vi "main_v20.vi"() -> ()   [LabVIEW 2016]
uses:
  <vilib>/Utility/file.llb/Write Delimited Spreadsheet (DBL).vi
  <vilib>/addons/database/Connection.llb/DB Tools Open Connec (Path).vi
  <vilib>/addons/database/Auxilliary.llb/DB Tools Format Datetime String (Time Stamp).vi
  <vilib>/addons/database/NI_Database_API.lvlib
panel:
  out "error out":errorcluster={"status"=FALSE, "code"=1073676418, "source"="VISA Close in N5700 Close.vi->main_v17.vi"}
  in  "Tab Control":T1(tab)
  out "Status_output_DC 2":bool caption="Ligado"
  out "Status_PS":bool caption="Conexão"
  out "Status_output_DC":bool caption="Ligado"
  out "Status_DC":bool caption="Conexão"
  out "battery_name 3":string="Manual" caption="Bateria Selecionada"
  in  "Historic_page":bool
  in  "graph_page":bool
  in  "Battery_page":bool
  in  "Test_page":bool
  in  "Charge_page":bool
  in  "Exit1":bool
  in  "Cap_nom":dbl caption="Capacidade Nominal (Ah)"
  in  "padrao_cap":dbl caption="Padrão Capacidade (h)"
  in  "Tensao_carga":dbl caption="Tensão Carga (V)"
  in  "corrente_res":dbl caption="Corrente Residual (A)"
  in  "SOC":dbl caption="Estado de Carga (%)"
  in  "corrente_max":dbl caption="Corrente de Carga (A)"
  in  "Tensao_corte":dbl caption="Tensão de Corte (V)"
  in  "ok_refresh_soc":bool
  in  "refresh_soc":bool
  in  "Charge_page2":bool
  in  "Test_page2":bool
  in  "New_battery":bool
  in  "Exit2":bool
  in  "Home1":bool
  out "data bateria":string[][](table)
  in  "Ativar Banco":bool
  in  "Table ID":u16(ring) items=["Bateria Unipower 1", "Bateria Unipower 2", "Bateria Unipower 3", "Bateria Unipower 4", "Bateria Unipower 5", "Bateria Unipower 6", "Bateria Unipower 7", "Bateria Unipower 8", "Bateria Litio 3 em serie"]
  in  "data_soc":cluster{"soc_db":dbl}={"soc_db"=100.0}
  in  "data insert":T2={"Descrição"="Descrição", "cap_db"=0.0, "tensao_nom_db"=0.0, "tensao_carg_db"=0.0, "corr_carg_db 2"=0.0, "tensao_corte_db"=0.0, "corr_res_db"=0.0, "soc_db"=0.0}
  in  "Exit3":bool
  in  "Home3":bool
  in  "Insert_battery":bool
  in  "Table ID 3":u16(ring) items=["Capacidade Nominal (Ah)", "Resistência Interna (ohm)", "Corrente de Curto-Circuito (A)"]
  in  "Table ID 2":u16(ring) items=["Bateria Unipower 1", "Bateria Unipower 2", "Bateria Unipower 3", "Bateria Unipower 4", "Bateria Unipower 5", "Bateria Unipower 6", "Bateria Unipower 7", "Bateria Unipower 8", "Bateria Litio 3 em serie"]
  out "data ensaio":string[][](table)
  in  "Exit4":bool
  in  "Home2":bool
  out "data bateria 2":string[][](table)
  in  "battery_select":bool
  in  "graph_select":bool
  in  "Exit5":bool
  in  "Home4":bool
  out "SoC_charge":dbl caption="Estado de Carga"
  out "Timer_charge":dbl caption="Tempo"
  out "Output_Current":dbl caption="Corrente"
  out "Output_Voltage":dbl caption="Tensão"
  out "Charge Active":bool
  in  "Radio Buttons":enum32{"Carga TC", "Carga CC"}(radio) caption="Modo de Carga"
  out "Current_Limit":dbl caption="Corrente"
  out "Voltage_Limit":dbl caption="Tensão"
  in  "Output On (T)":bool
  in  "auxiliar 2":bool
  out "battery_name 2":string="Manual" caption="Bateria Selecionada"
  out "soc_ensaio":dbl caption="Estado de Carga"
  out "Timer_ensaio":dbl caption="Tempo"
  out "DC_Current":dbl caption="Corrente"
  out "DC_Voltage":dbl caption="Tensão"
  in  "Start":bool
  out "CC Active":bool
  in  "battery_select2":bool
  in  "graph_select2":bool
  out "battery_name":string="Manual" caption="Bateria Selecionada"
  in  "Ensaios":u16(ring) items=["Capacidade Regime Nominal", "Capacidade Diferente de Regime Nominal", "Resistência Interna", "Ciclos de carga e descarga", "Caracterização"]
  in  "Exit6":bool
  in  "cap_soc":dbl caption="Capacidade"
  in  "info_ensaio":enum32{"1", "2", "3", "4", "5"}(tab)
  out "padrao_cap2":dbl caption="Padrão Capacidade (h)"
  out "cap_bat":dbl caption="Capacidade (Ah)"
  out "cap_nom_ensaio":dbl caption="Capacidade Real (Ah)"
  in  "aux_cap_ensaio":bool
  in  "aux_soc_ensaio1":bool
  out "cap_fn_calc":dbl caption="Capacidade Real (Ah)"
  in  "cap_fn":dbl caption="Capacidade (Ah)"
  in  "corr_fn":dbl caption="Corrente (A)"
  out "res_cap":dbl caption="Capacidade (Ah)"
  out "res_ensaio":dbl caption="Resistência (ohm)"
  out "curto_ensaio":dbl caption="Corrente Curto-Circuito (A)"
  out "res_volt_1":dbl caption="Volt_res_1"
  out "res_curr_1":dbl caption="Corr_res_1"
  out "res_curr_2":dbl caption="Corr_res_2"
  out "res_volt_2":dbl caption="Volt_res_2"
  in  "aux_res_ensaio":bool
  in  "aux_soc_ensaio2":bool
  in  "curr_carac":dbl caption="Corrente"
  in  "twait":dbl caption="Tempo Relax"
  in  "cap_caract":dbl caption="Capacidade"
  in  "pulso_soc":dbl caption="Pulso SoC"
  out "cont_pulso":dbl caption="Contador Pulso"
  out "est_time":dbl caption="Tempo Estimado"
  out "COP":bool
  in  "tinicio":dbl caption="T inicio"
  out "tpulso":dbl caption="Tempo Descarga"
  in  "Home5":bool
  out "cap_ensaio":dbl caption="Capacidade"
  in  "aux_soc":bool
  out "WFC Current Load":dbl(graph)=0.007083870470523834
  out "WFC Voltage Load":dbl(graph)=12.54011344909668
  out "Waveform Chart Voltage":dbl(graph)=12.56
  out "Waveform Chart Current":dbl(graph)
  in  "back_charge":bool
  in  "back_ens":bool
  in  "Home6":bool
  in  "Exit7":bool
  # "MENU"
  # "Desenvolvido por William Rocha"
  # "Deseja ativar o banco de dados?"
  # "BATERIAS"
  # "Desenvolvido por William Rocha"
  # "REGISTRAR BATERIA"
  # "Desenvolvido por William Rocha"
  # "Desenvolvido por William Rocha"
  # "MOSTRAR BATERIAS"
  # "Instruções"
  # "Para iniciar o ensaio de capacidade siga o procedimento de abaixo:\n  1 - Verifique se a bateria está conectada aos equipamentos  \n  2 - Verifique a bateria selecionada no banco de dados ou insira os dados manualmente  \n  3 - Selecione o modo de carga\n  4 - Pressione o botão iniciar carga\n\n  A carga é finalizada ao atingir 100 % do estado de carga. A carga pode ser encerrada em qualquer momento pelo usuário da carga."
  # "Desenvolvido por William Rocha"
  # "RECARGA"
  # "V"
  # "A"
  # "%"
  # "s"
  # "Iniciar Carga"
  # "Configuração"
  # "V"
  # "A"
  # "Modo de  Carga"
  # "Medições"
  # "Iniciar Ensaio"
  # "Medições"
  # "V"
  # "A"
  # "Ensaio Ativo"
  # "%"
  # "s"
  # "Instruções"
  # "Para iniciar o ensaio siga o procedimento de abaixo:\n  1 - Verifique se a bateria está conectada aos equipamentos\n  2 - Verifique a bateria selecionada no banco de dados ou insira os dados manualmente \n  3 - Pressione o botão iniciar carga\n  4 - Espere até o fim do ensaio para obter o resultado\n\n  O ensaio é finalizado automaticamente e o resultado será inserido no banco de dados, caso o mesmo esteja ativado. Porém, o ensaio pode ser encerrado em qualquer momento pelo usuário e o resultado não será contabalizado."
  # "ENSAIOS"
  # "Desenvolvido por William Rocha"
  # "Fonte CC"
  # "Carga Eletrônica"
  # "Desenvolvido por William Rocha"
  # "Gráficos"
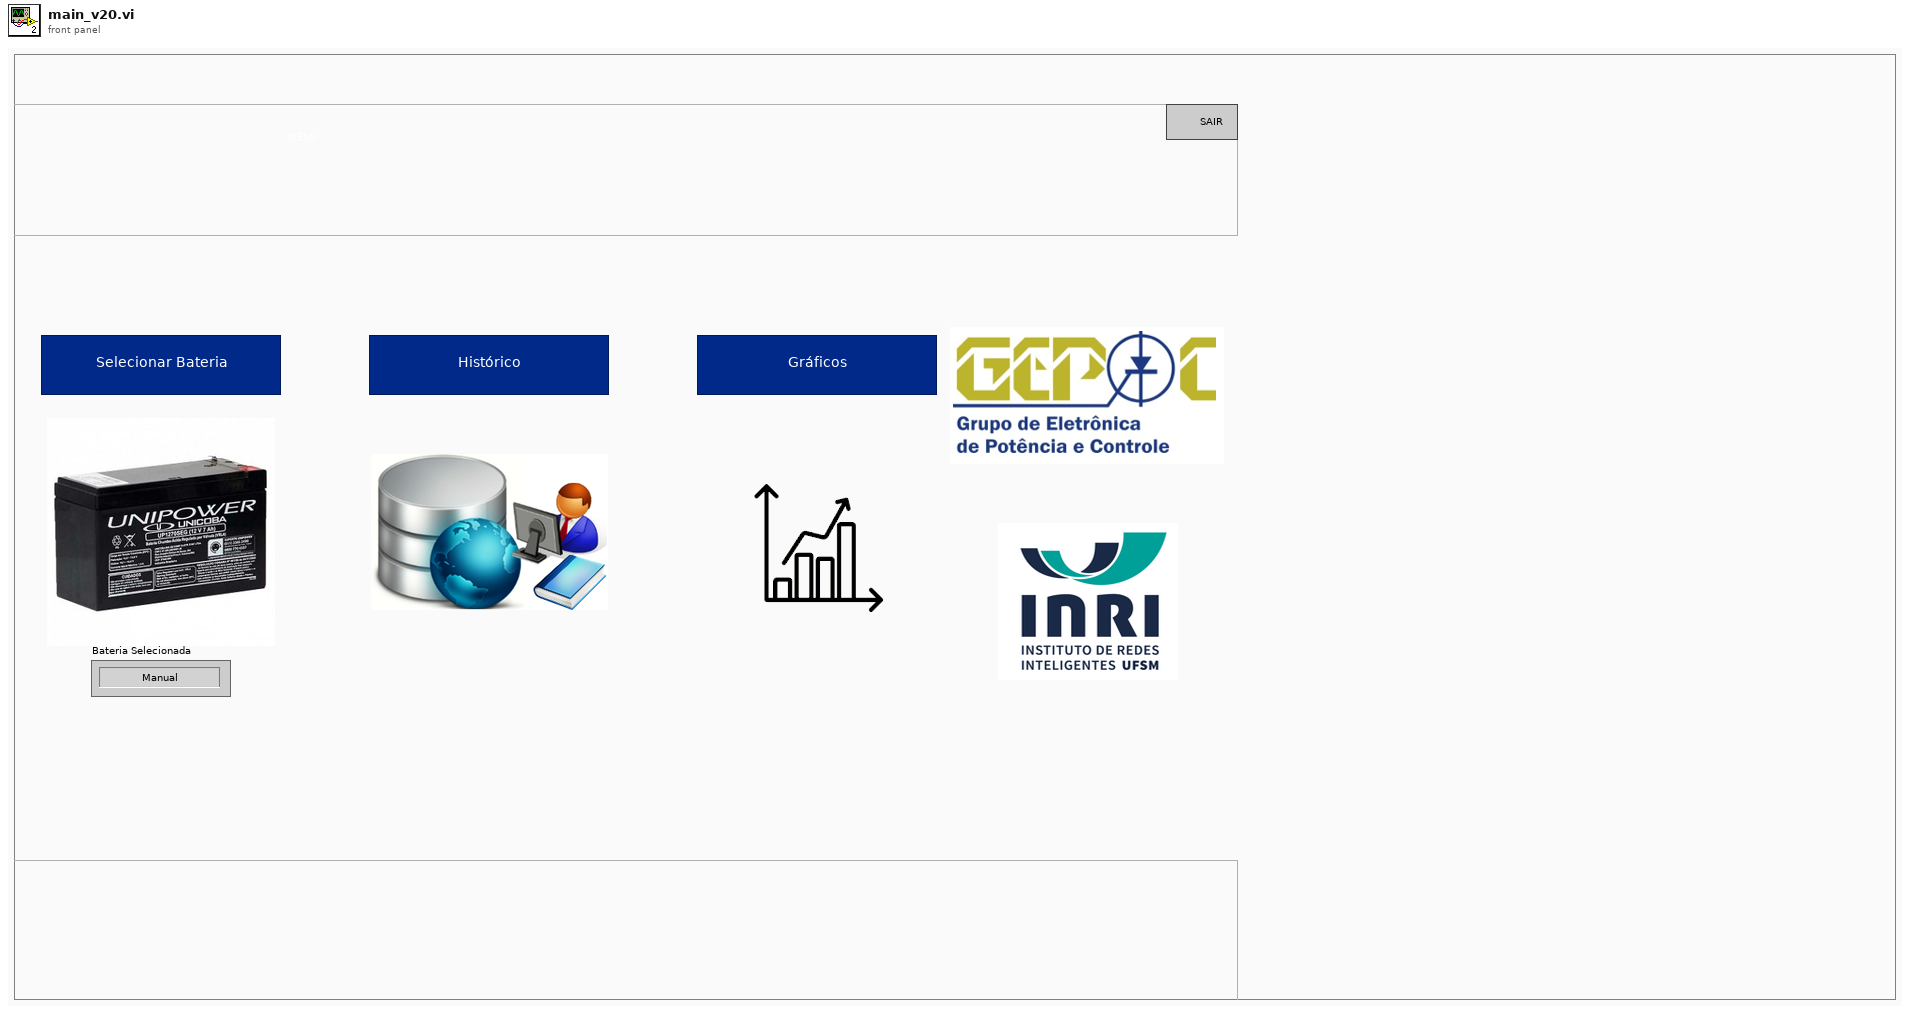
[diagram p1: front panel]
types:
  T1 = enum32{"Home", "Battery Page", "Register Battery Page", "Show battery page", "Charge Page", "Test Page", "Graphs"}
  T2 = cluster{"Descrição":string, "cap_db":dbl, "tensao_nom_db":dbl, "tensao_carg_db":dbl, "corr_carg_db 2":dbl, "tensao_corte_db":dbl, "corr_res_db":dbl, "soc_db":dbl}
  T3 = enum32{"Home", "Battery Page", "Register Battery Page", "Show battery page", "Charge Page", "Test Page"}
  T4 = typedef "NI_Database_API.lvlib/Conn ObjectReference.ctl" = refnum<k1>
  T5 = cluster{"Table ID":u16, "date/time string":string, i32, "cap_nom_ensaio":dbl}
  T6 = cluster{"Table ID":u16, "date/time string":string, i32, "res_ensaio":dbl}
  T7 = cluster{"Table ID":u16, "date/time string":string, i32, "curto_ensaio":dbl}
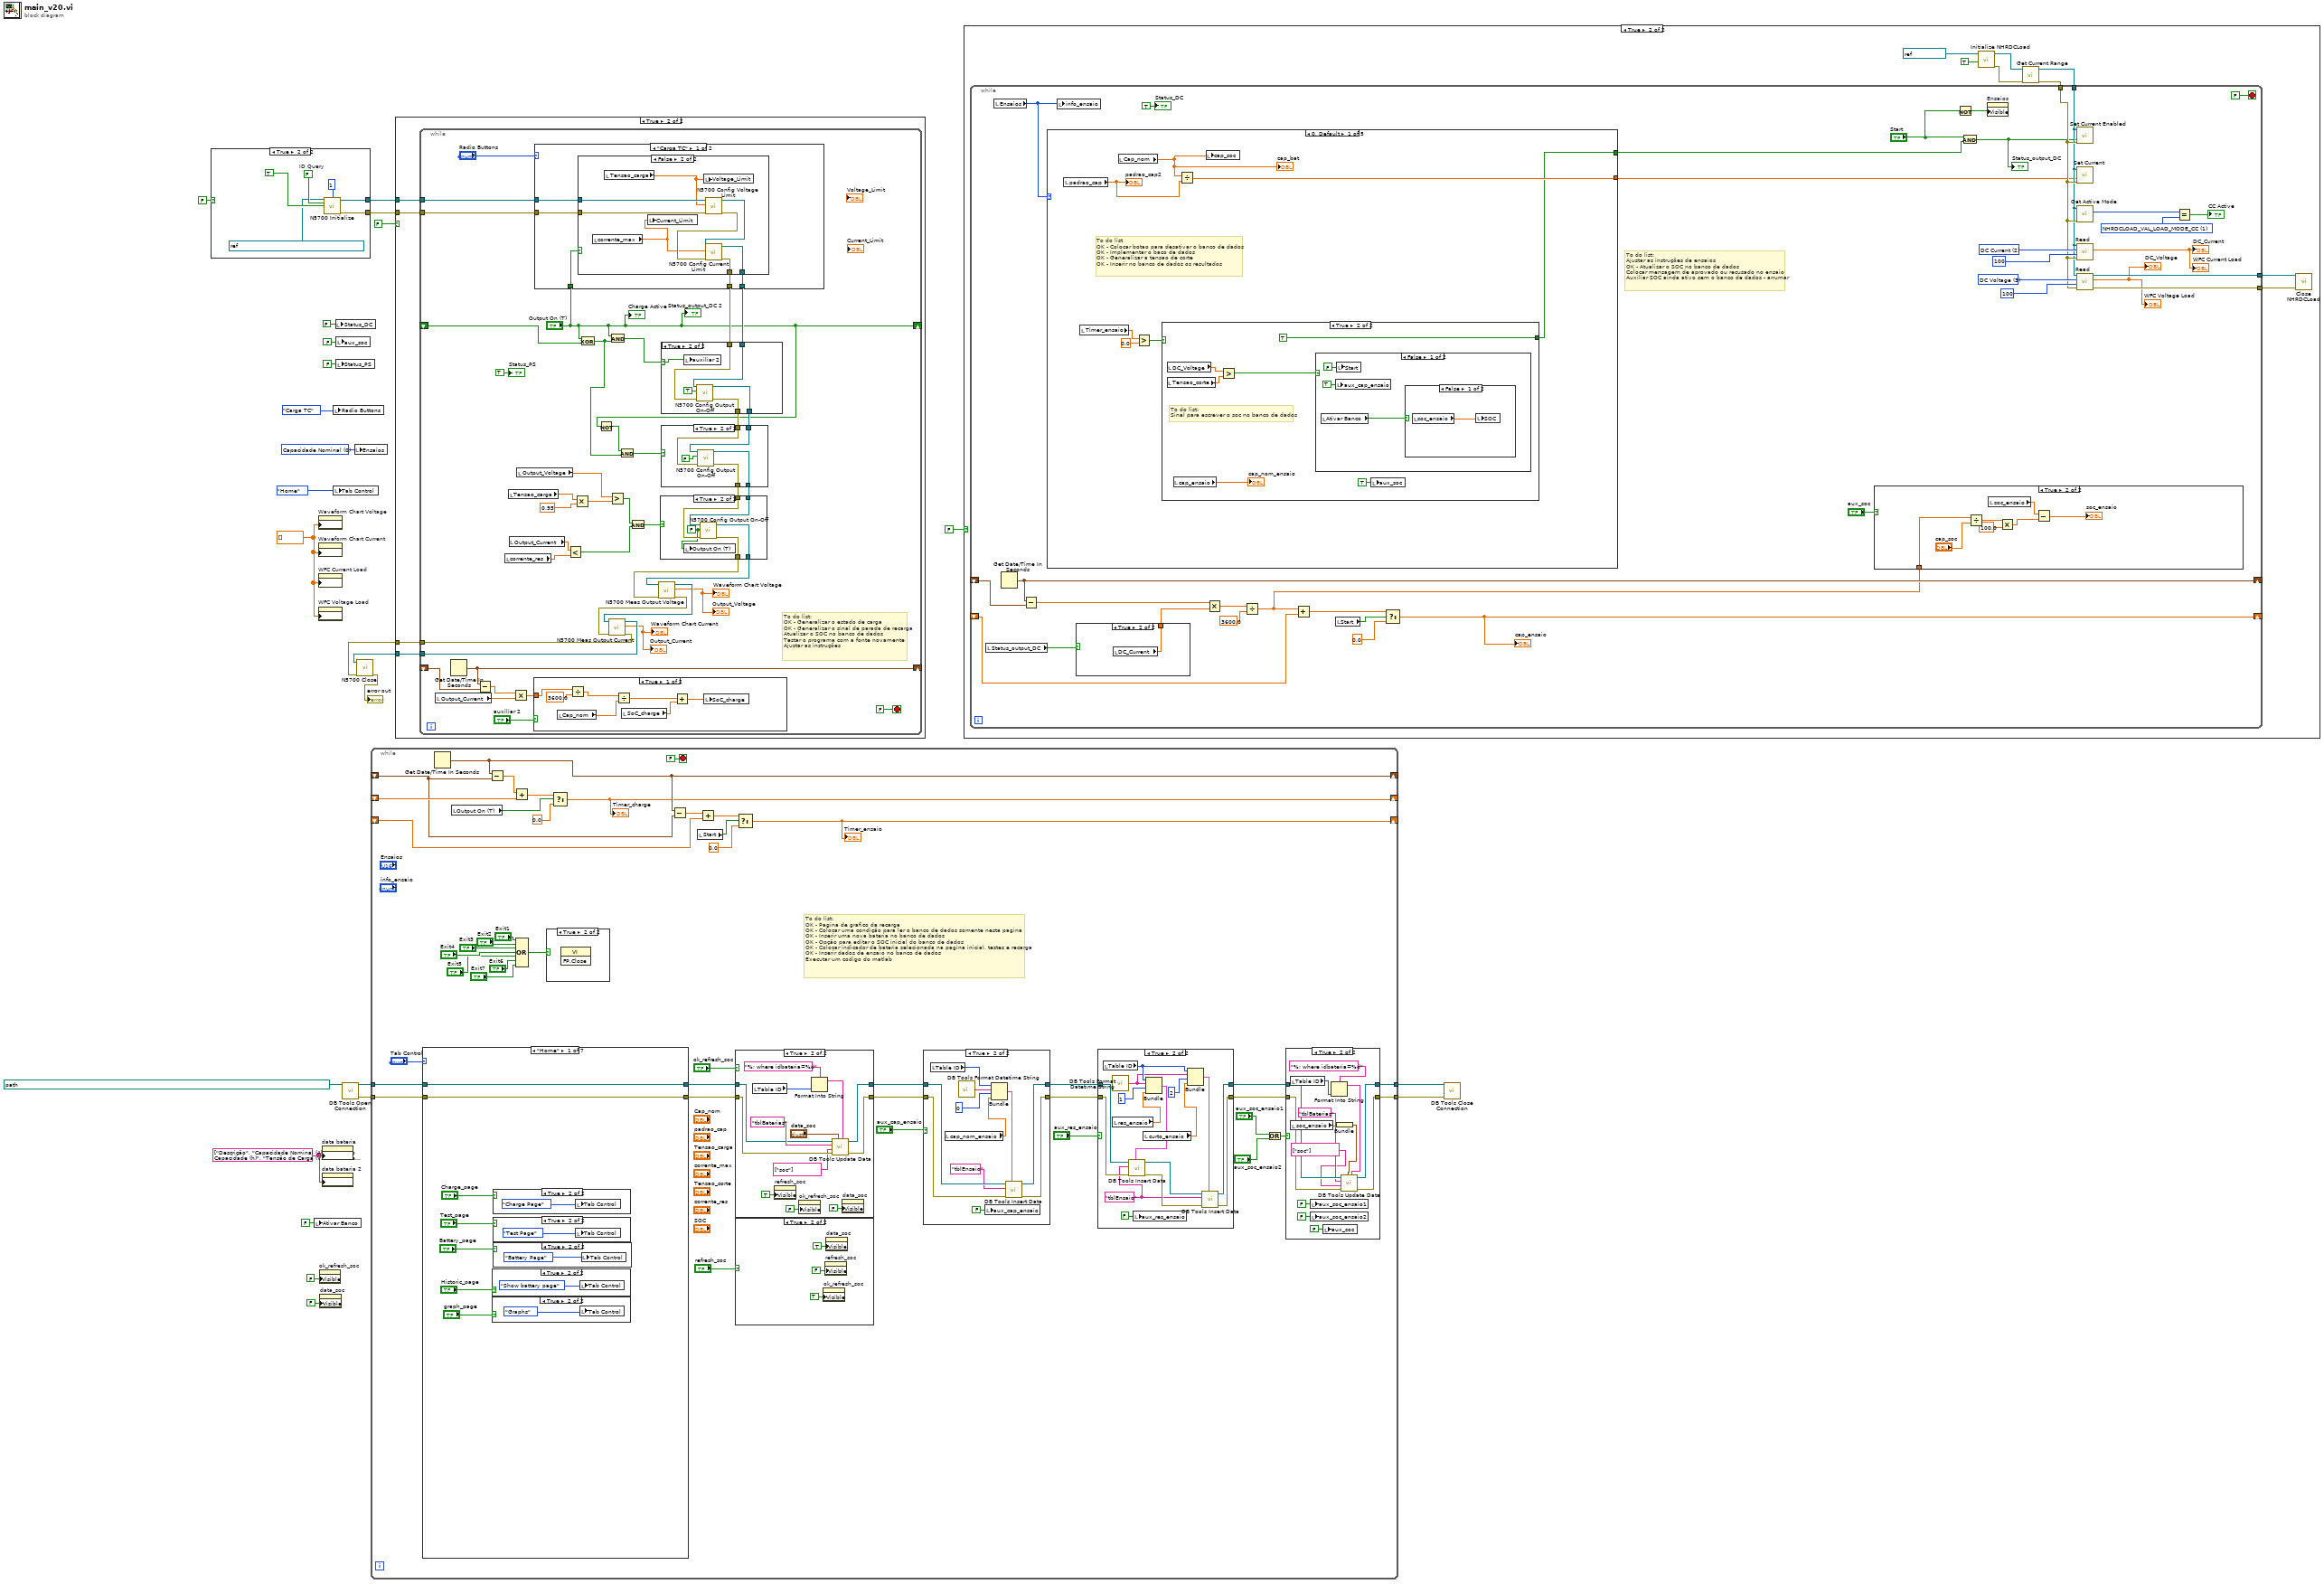
[diagram p0: block diagram]
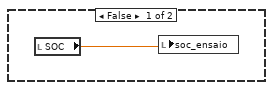
[diagram p4: hidden frame]
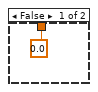
[diagram p5: hidden frame]
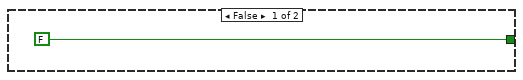
[diagram p6: hidden frame]
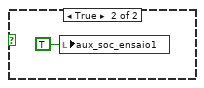
[diagram p7: hidden frame]
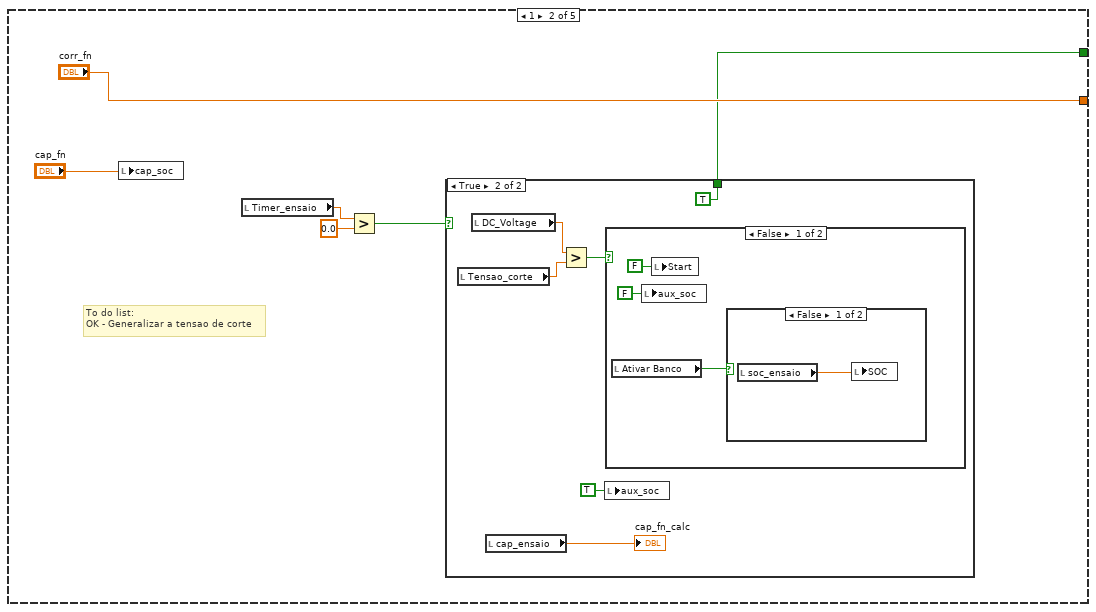
[diagram p9: hidden frame]
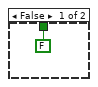
[diagram p10: hidden frame]
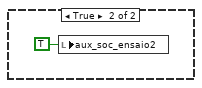
[diagram p11: hidden frame]
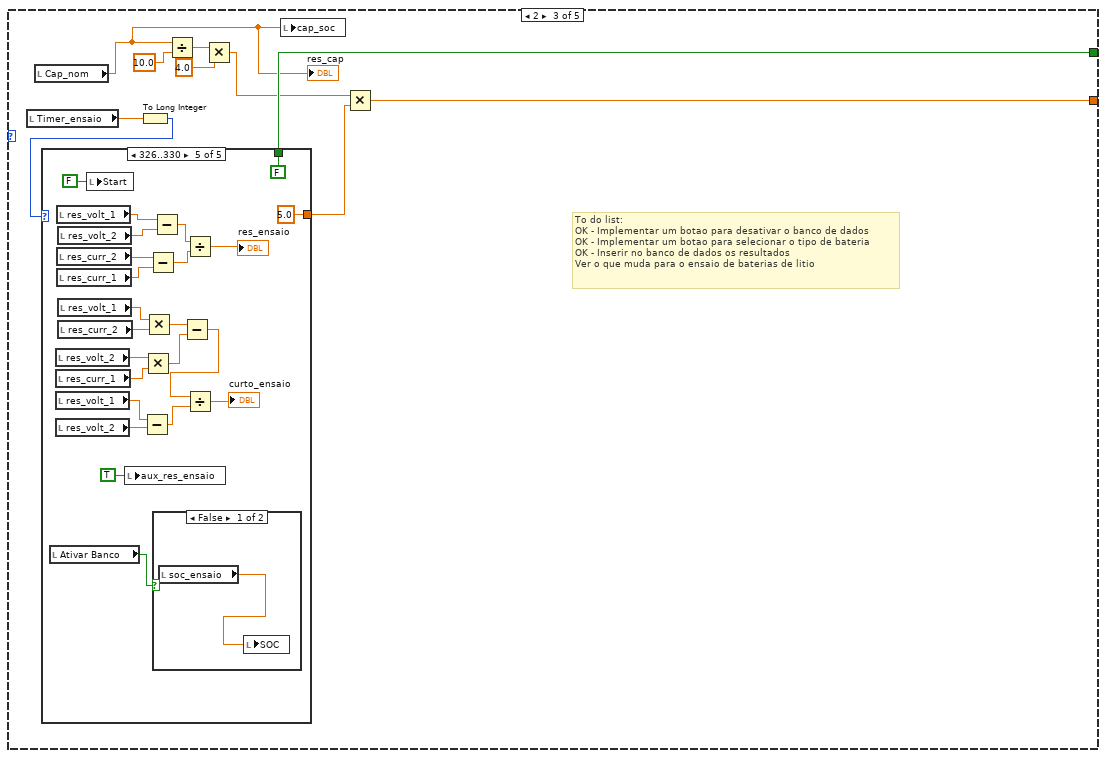
[diagram p13: hidden frame]
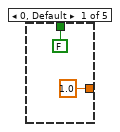
[diagram p14: hidden frame]
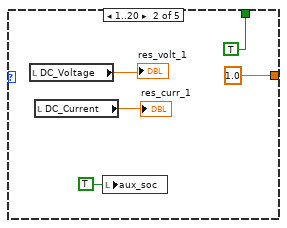
[diagram p15: hidden frame]
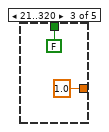
[diagram p16: hidden frame]
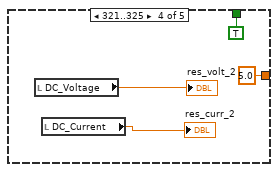
[diagram p17: hidden frame]
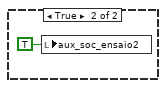
[diagram p18: hidden frame]
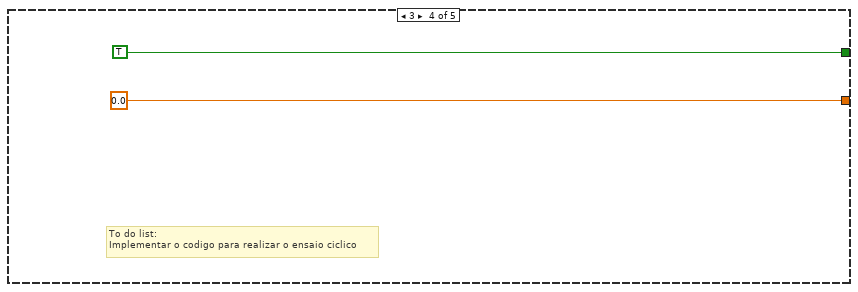
[diagram p19: hidden frame]
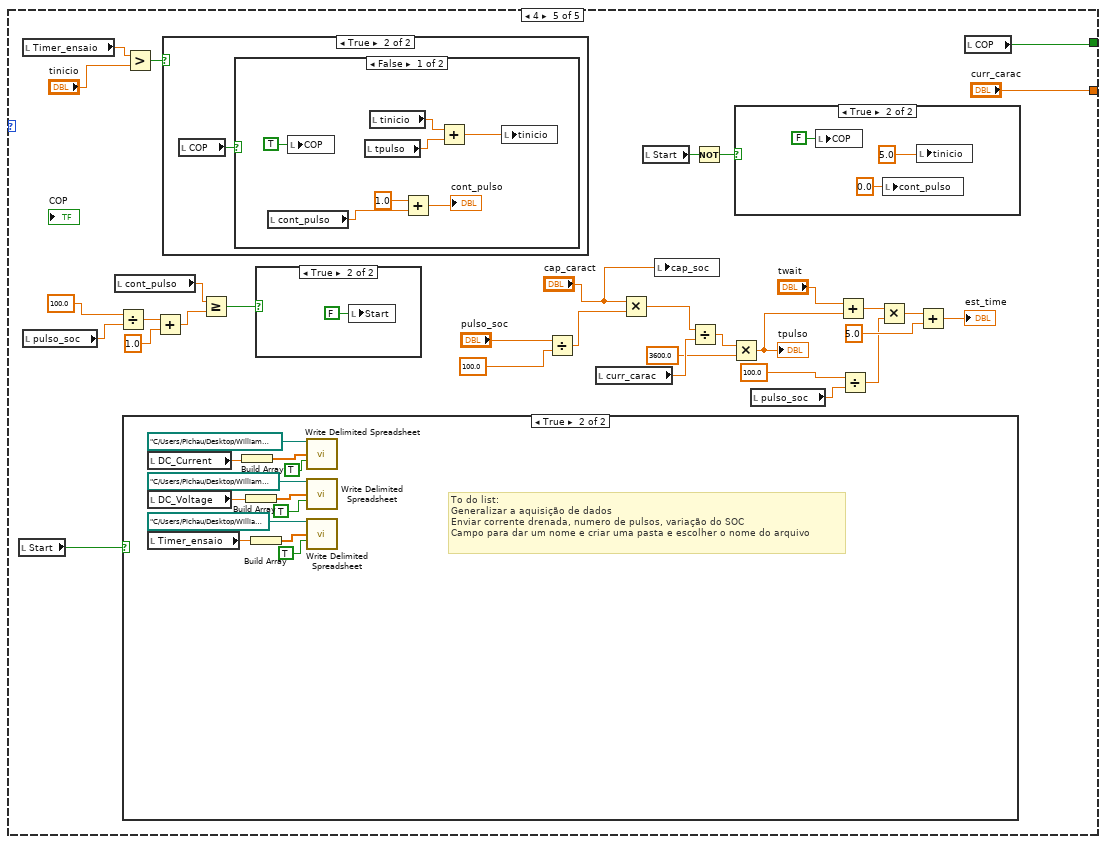
[diagram p20: hidden frame]
diagram:
  w6 = string[] ["Descrição", "Capacidade Nominal (Ah)", "Padrão Capacidade (h)", "Tensão de Carga (V)", "Corrente Máxima (A)", "Tensão de Corte (V)", "Corrente Residual (A)", "SOC (%)"] ("columns")
  w14 = u16 0 items=["Capacidade Nominal"] ("Table ID")
  w10 = dbl[] [] ("History Data")
  n1 = case shown="True" FALSE {
    tunnel: [_ w25] -> w23
    tunnel: [_ w27] -> w20
    frame False {
    }
    frame True {
      w29 = FALSE  # ID Query
      n2 = call <instrlib>:"N5700 Initialize.vi"("VISA name"=refnum<visa-resource-name> "TCPIP0::A-N8762A-1651P.local::inst0::INSTR", "Timeout (3 sec)"=u32 1, "ID Query (T)"=w29, "Reset (T)"=TRUE ("Reset (F)")) -> ("VISA out"=w25:refnum<visa-resource-name>, "error out"=w27:errorcluster)  [unwired: 10 in]
    }
  }
  n3 = local write "Ativar Banco"(FALSE ("Ativar Banco")) -> ()
  n4 = property on="Waveform Chart Voltage" class="WFChart (strict)"("History Data"=w10) -> ()  [unwired: 2 in, 2 out]
  n5 = property on="Waveform Chart Current" class="WFChart (strict)"("History Data"=w10) -> ()  [unwired: 2 in, 2 out]
  n6 = property on="WFC Current Load" class="WFChart (strict)"("History Data"=w10) -> ()  [unwired: 2 in, 2 out]
  n7 = property on="WFC Voltage Load" class="WFChart (strict)"("History Data"=w10) -> ()  [unwired: 2 in, 2 out]
  n8 = property on="ok_refresh_soc" class="Bool"("Visible"=FALSE) -> ()  [unwired: 2 in, 2 out]
  n9 = property on="data_soc" class="Clust (strict)"("Visible"=FALSE) -> ()  [unwired: 2 in, 2 out]
  n10 = property on="data bateria" class="Tbl (strict)"("Column Headers[]"=w6) -> ()  [unwired: 2 in, 2 out]
  n11 = property on="data bateria 2" class="Tbl (strict)"("Column Headers[]"=w6) -> ()  [unwired: 2 in, 2 out]
  n12 = local write "Radio Buttons"(enum32{"Carga TC", "Carga CC"}."Carga TC" ("Radio Buttons")) -> ()
  n13 = local write "Tab Control"(T3."Home" ("Tab Control")) -> ()
  n14 = local write "Status_DC"(FALSE ("Status_DC")) -> ()
  n15 = local write "aux_soc"(FALSE ("aux_soc")) -> ()
  n16 = local write "Status_PS"(FALSE ("Status_PS")) -> ()
  n17 = call-poly <vilib>:"DB Tools Open Connection.vi"("connection information"=path "D:/UFSM/Engenharia de Controle e Automação/9 Semestre/Trabalho de Conclusão de Curso “A” – DPEE 1046/TCC/TCC - William Rochav5/database/database2_2.udl") -> ("error out"=w7:errorcluster, "connection reference"=w8:T4)  [unwired: 7 in]
  n18 = local write "Ensaios"(w14) -> ()
  n19 = while {
    shift-right: [w66] -> _
    shift-left: _ -> [w65]
    shift-right: [w59] -> _
    shift-left: _ -> [w72]
    shift-right: [w58] -> _
    shift-left: _ -> [w61]
    tunnel: w8 -> [w49]
    tunnel: w7 -> [w48]
    tunnel: [w37] -> w5
    tunnel: [w35] -> w4
    stop <- FALSE stop-if-true
    # "To do list:\nOK - Pagina de grafico da recarga\nOK - Colocar uma condição para ler o banco de dados somente nesta pagina\nOK - Inserir uma nova bateria no banco de dados\nOK - Opção para editar o SOC inicial do banco de dados\nOK - Colocar indicador de bateria selecionada na pagina inicial, testes e recarga\nOK - Inserir dados de ensaio no banco de dados\nExecutar um codigo do matlab"
    n20 = case shown="\"Home\"" "Tab Control" {
      tunnel: [w140 w157 w216 w236 w254 w262 w270] -> w47
      tunnel: w49 -> [w140 w160 w217 w239 w254 w262 w270]
      tunnel: [w139 w158 w215 w237 w253 w261 w269] -> w46
      tunnel: w48 -> [w139 w159 w218 w238 w253 w261 w269]
      frame "Home" {
        n21 = case shown="True" "Historic_page" {
          frame False {
          }
          frame True {
            n22 = local write "Tab Control"(T3."Show battery page" ("Tab Control")) -> ()
          }
        }
        n23 = case shown="True" "graph_page" {
          frame False {
          }
          frame True {
            n24 = local write "Tab Control"(T1."Graphs" ("Tab Control")) -> ()
          }
        }
        n25 = case shown="True" "Charge_page" {
          frame False {
          }
          frame True {
            n26 = local write "Tab Control"(T3."Charge Page" ("Tab Control")) -> ()
          }
        }
        n27 = case shown="True" "Test_page" {
          frame False {
          }
          frame True {
            n28 = local write "Tab Control"(T3."Test Page" ("Tab Control")) -> ()
          }
        }
        n29 = case shown="True" "Battery_page" {
          frame False {
          }
          frame True {
            n30 = local write "Tab Control"(T3."Battery Page" ("Tab Control")) -> ()
          }
        }
      }
      frame "Battery Page" {
        n31 = Not(x="Ativar Banco") -> (.not. x?=w151:bool)
        n32 = case shown="True" "Ativar Banco" {
          tunnel: w160 -> [w171 w207]
          tunnel: w159 -> [w170 w206]
          tunnel: [w171 w203] -> w157
          tunnel: [w170 w202] -> w158
          frame False {
            w166 = FALSE ("Visible")
            w169 = "Manual" ("battery_name")
            n33 = property on="New_battery" class="Bool"("Visible"=FALSE) -> ()  [unwired: 2 in, 2 out]
            n34 = property on="data_soc" class="Clust (strict)"("Visible"=w166) -> ()  [unwired: 2 in, 2 out]
            n35 = property on="refresh_soc" class="Bool"("Visible"=FALSE) -> ()  [unwired: 2 in, 2 out]
            n36 = property on="ok_refresh_soc" class="Bool"("Visible"=FALSE) -> ()  [unwired: 2 in, 2 out]
            n37 = property on="Table ID" class="Ring (strict)"("Visible"=w166) -> ()  [unwired: 2 in, 2 out]
            "battery_name" <- w169
            "battery_name 2" <- w169
            "battery_name 3" <- w169
          }
          frame True {
            w173 = TRUE ("Visible")
            n38 = call <vilib>:"DB Tools Select All Data.vi"("error in (no error)"=w206, "columns"=string[] ["Descricao", "capacidade", "padrao_cap", "tensao_carga", "corrente", "tensao_corte", "corrente_res", "soc"], "table"="tblBaterias", "connection reference"=w207) -> ("error out"=w202:errorcluster, "data"=w177:string[][], "connection reference out"=w203:T4)  [unwired: 2 in]
            "data bateria" <- w177
            n39 = Index Array(array=w177, index (row)="Table ID", index (col)=1 ("disabled index (col)")) -> (element=w199:string)
            n40 = Index Array(array=w177, index (row)="Table ID", index (col)=2) -> (element=w194:string)
            n41 = Index Array(array=w177, index (row)="Table ID", index (col)=3) -> (element=w193:string)
            n42 = Index Array(array=w177, index (row)="Table ID", index (col)=4 ("disabled index (col)")) -> (element=w183:string)
            n43 = Index Array(array=w177, index (row)="Table ID", index (col)=5 ("disabled index (col)")) -> (element=w184:string)
            n44 = Index Array(array=w177, index (row)="Table ID", index (col)=6 ("disabled index (col)")) -> (element=w185:string)
            n45 = Index Array(array=w177, index (row)="Table ID", index (col)=7 ("disabled index (col)")) -> (element=w186:string)
            n46 = Index Array(array=w177, index (row)="Table ID", index (col)=0 ("disabled index (col)")) -> (element=w174:string)
            n47 = Fract/Exp String To Number(use system decimal point (T)=TRUE, string=w199) -> (number=w197:dbl)  [unwired: 2 in, 1 out]
            n48 = Fract/Exp String To Number(string=w194) -> (number=w192:dbl)  [unwired: 3 in, 1 out]
            n49 = Fract/Exp String To Number(string=w193) -> (number=w191:dbl)  [unwired: 3 in, 1 out]
            n50 = Fract/Exp String To Number(string=w183) -> (number=w182:dbl)  [unwired: 3 in, 1 out]
            n51 = Fract/Exp String To Number(string=w184) -> (number=w181:dbl)  [unwired: 3 in, 1 out]
            n52 = Fract/Exp String To Number(string=w185) -> (number=w179:dbl)  [unwired: 3 in, 1 out]
            n53 = Fract/Exp String To Number(string=w186) -> (number=w180:dbl)  [unwired: 3 in, 1 out]
            n54 = local write "battery_name"(w174) -> ()
            n55 = local write "battery_name 2"(w174) -> ()
            n56 = local write "battery_name 3"(w174) -> ()
            n57 = local write "Tensao_carga"(w191) -> ()
            n58 = local write "corrente_max"(w182) -> ()
            n59 = local write "Tensao_corte"(w181) -> ()
            n60 = local write "Cap_nom"(w197) -> ()
            n61 = local write "padrao_cap"(w192) -> ()
            n62 = local write "corrente_res"(w179) -> ()
            n63 = local write "SOC"(w180) -> ()
            n64 = Index Array(array=w177, index (col)=0) -> (element=w201:string[])  [unwired: 1 in]
            n65 = property on="refresh_soc" class="Bool"("Visible"=w173) -> ()  [unwired: 2 in, 2 out]
            n66 = property on="New_battery" class="Bool"("Visible"=TRUE) -> ()  [unwired: 2 in, 2 out]
            n67 = property on="Table ID" class="Ring (strict)"("Visible"=w173) -> ()  [unwired: 2 in, 2 out]
            n68 = property on="Table ID" class="Ring (strict)"("Strings []"=w201) -> ()  [unwired: 2 in, 2 out]
            n69 = property on="Table ID 2" class="Ring (strict)"("Strings []"=w201) -> ()  [unwired: 2 in, 2 out]
          }
        }
        n70 = property on="data bateria" class="Tbl (strict)"("Visible"="Ativar Banco") -> ()  [unwired: 2 in, 2 out]
        n71 = property on="Cap_nom" class="DigNum (strict)"("Visible"=w151) -> ()  [unwired: 2 in, 2 out]
        n72 = property on="padrao_cap" class="DigNum (strict)"("Visible"=w151) -> ()  [unwired: 2 in, 2 out]
        n73 = property on="Tensao_carga" class="DigNum (strict)"("Visible"=w151) -> ()  [unwired: 2 in, 2 out]
        n74 = property on="corrente_max" class="DigNum (strict)"("Visible"=w151) -> ()  [unwired: 2 in, 2 out]
        n75 = property on="Tensao_corte" class="DigNum (strict)"("Visible"=w151) -> ()  [unwired: 2 in, 2 out]
        n76 = property on="corrente_res" class="DigNum (strict)"("Visible"=w151) -> ()  [unwired: 2 in, 2 out]
        n77 = property on="SOC" class="DigNum (strict)"("Visible"=w151) -> ()  [unwired: 2 in, 2 out]
        n78 = case shown="True" "New_battery" {
          frame False {
          }
          frame True {
            n79 = local write "Tab Control"(T3."Register Battery Page" ("Tab Control")) -> ()
          }
        }
        n80 = case shown="True" "Charge_page2" {
          frame False {
          }
          frame True {
            n81 = local write "Tab Control"(T3."Charge Page" ("Tab Control")) -> ()
          }
        }
        n82 = case shown="True" "Test_page2" {
          frame False {
          }
          frame True {
            n83 = local write "Tab Control"(T3."Test Page" ("Tab Control")) -> ()
          }
        }
        n84 = case shown="True" "Home1" {
          frame False {
          }
          frame True {
            n85 = local write "Tab Control"(T3."Home" ("Tab Control")) -> ()
          }
        }
      }
      frame "Show battery page" {
        n86 = local read "Table ID 3"() -> (w210:u16)
        n87 = property on="Table ID 3" class="Ring (strict)"() -> ("Strings []"=w209:string[])  [unwired: 2 in, 2 out]
        n88 = Index Array(array=w209, index=w210) -> (element=w211:string)
        n89 = case shown="True" "Home2" {
          frame False {
          }
          frame True {
            n90 = local write "Tab Control"(T3."Home" ("Tab Control")) -> ()
          }
        }
        n91 = call <vilib>:"DB Tools Select All Data.vi"("error in (no error)"=w218, "columns"=string[] ["Descricao", "capacidade", "padrao_cap", "tensao_carga", "corrente", "tensao_corte", "corrente_res", "soc"], "table"="tblBaterias", "connection reference"=w217) -> ("error out"=w222:errorcluster, "data"=→"data bateria 2":string[][], "connection reference out"=w221:T4)  [unwired: 2 in]
        n92 = Format Into String(format string="%; where idbateria=%d" ("condition"), "Table ID 2") -> (resulting string=w230:string)  [unwired: 2 in, 1 out]
        n93 = Format Into String(format string="%; and tipo=%d" ("condition"), "Table ID 3") -> (resulting string=w229:string)  [unwired: 2 in, 1 out]
        n94 = Insert Into Array(array=string[] ["Data"], index=1, new element=w211) -> (w214:string[])
        n95 = Concatenate Strings(w230, w229) -> (w231:string)
        n96 = call <vilib>:"DB Tools Select All Data.vi"("optional clause"=w231, "error in (no error)"=w222, "columns"=string[] ["data_ensaio", "valor"], "table"="tblEnsaio", "connection reference"=w221) -> ("error out"=w215:errorcluster, "data"=→"data ensaio":string[][], "connection reference out"=w216:T4)  [unwired: 1 in]
        n97 = property on="data ensaio" class="Tbl (strict)"("Column Headers[]"=w214) -> ()  [unwired: 2 in, 2 out]
      }
      frame "Register Battery Page" {
        n98 = case shown="True" "Home3" {
          frame False {
          }
          frame True {
            n99 = local write "Tab Control"(T3."Home" ("Tab Control")) -> ()
          }
        }
        n100 = case shown="True" "Insert_battery" {
          tunnel: w239 -> [w242 w249]
          tunnel: w238 -> [w241 w248]
          tunnel: [w241 w247] -> w237
          tunnel: [w242 w246] -> w236
          frame False {
          }
          frame True {
            n101 = call <vilib>:"DB Tools Insert Data.vi"("data"="data insert", "error in (no error)"=w248, "table"="tblBaterias", "connection reference"=w249) -> ("error out"=w247:errorcluster, "connection reference out"=w246:T4)  [unwired: 6 in]
            n102 = local write "Tab Control"(T1."Battery Page" ("Tab Control")) -> ()
          }
        }
      }
      frame "Charge Page" {
        n103 = case shown="True" "Home4" {
          frame False {
          }
          frame True {
            n104 = local write "Tab Control"(T3."Home" ("Tab Control")) -> ()
          }
        }
        n105 = case shown="True" "battery_select" {
          frame False {
          }
          frame True {
            n106 = local write "Tab Control"(T1."Battery Page" ("Tab Control")) -> ()
          }
        }
        n107 = case shown="True" "graph_select" {
          frame False {
          }
          frame True {
            n108 = local write "Tab Control"(T1."Graphs" ("Tab Control")) -> ()
          }
        }
      }
      frame "Graphs" {
        n109 = case shown="True" "back_charge" {
          frame False {
          }
          frame True {
            n110 = local write "Tab Control"(T1."Charge Page" ("Tab Control")) -> ()
          }
        }
        n111 = case shown="True" "back_ens" {
          frame False {
          }
          frame True {
            n112 = local write "Tab Control"(T1."Test Page" ("Tab Control")) -> ()
          }
        }
        n113 = case shown="True" "Home6" {
          frame False {
          }
          frame True {
            n114 = local write "Tab Control"(T1."Home" ("Tab Control")) -> ()
          }
        }
      }
      frame "Test Page" {
        n115 = case shown="True" "Home5" {
          frame False {
          }
          frame True {
            n116 = local write "Tab Control"(T3."Home" ("Tab Control")) -> ()
          }
        }
        n117 = case shown="True" "battery_select2" {
          frame False {
          }
          frame True {
            n118 = local write "Tab Control"(T1."Battery Page" ("Tab Control")) -> ()
          }
        }
        n119 = case shown="True" "graph_select2" {
          frame False {
          }
          frame True {
            n120 = local write "Tab Control"(T1."Graphs" ("Tab Control")) -> ()
          }
        }
      }
    }
    n121 = Get Date/Time In Seconds() -> (seconds since 1Jan1904=w66:timestamp)
    n122 = local read "Output On (T)"() -> (w67:bool)
    n123 = Subtract(x=w66, y=w65) -> (x-y=w73:dbl)
    n124 = Add(x=w73, y=w72) -> (x+y=w70:dbl)
    n125 = Compound Arithmetic op=OR("Exit1", "Exit2", "Exit3", "Exit4", "Exit5", "Exit6", "Exit7") -> (w56:bool)
    n126 = case shown="True" w56 {
      frame False {
      }
      frame True {
        n127 = invoke class="VI" method="FP.Close"() -> ()  [unwired: 3 in, 3 out]
      }
    }
    n128 = Select(t=w70, s=w67, f=0.0) -> (s? t:f=w59:dbl)
    "Timer_charge" <- w59
    n129 = Subtract(x=w66, y=w65) -> (x-y=w64:dbl)
    n130 = local read "Start"() -> (w62:bool)
    n131 = Add(x=w64, y=w61) -> (x+y=w63:dbl)
    n132 = case shown="True" "ok_refresh_soc" {
      tunnel: [w125 w138] -> w43
      tunnel: [w124 w137] -> w42
      tunnel: w47 -> [w125 w133]
      tunnel: w46 -> [w124 w134]
      frame False {
      }
      frame True {
        n133 = local read "Table ID"() -> (w131:u16)
        n134 = property on="refresh_soc" class="Bool"("Visible"=TRUE) -> ()  [unwired: 2 in, 2 out]
        n135 = property on="ok_refresh_soc" class="Bool"("Visible"=FALSE) -> ()  [unwired: 2 in, 2 out]
        n136 = Format Into String(format string="%; where idbateria=%d" ("condition"), w131) -> (resulting string=w130:string)  [unwired: 2 in, 1 out]
        n137 = call <vilib>:"DB Tools Update Data.vi"("condition"=w130, "data"="data_soc", "error in (no error)"=w134, "columns"=string[] ["soc"], "table"="tblBaterias", "connection reference"=w133) -> ("error out"=w137:errorcluster, "connection reference out"=w138:T4)  [unwired: 4 in]
        n138 = property on="data_soc" class="Clust (strict)"("Visible"=FALSE) -> ()  [unwired: 2 in, 2 out]
      }
    }
    n139 = case shown="True" "refresh_soc" {
      frame False {
      }
      frame True {
        n140 = property on="ok_refresh_soc" class="Bool"("Visible"=TRUE) -> ()  [unwired: 2 in, 2 out]
        n141 = property on="refresh_soc" class="Bool"("Visible"=FALSE) -> ()  [unwired: 2 in, 2 out]
        n142 = property on="data_soc" class="Clust (strict)"("Visible"=TRUE) -> ()  [unwired: 2 in, 2 out]
      }
    }
    n143 = Select(t=w63, s=w62, f=0.0) -> (s? t:f=w58:dbl)
    "Timer_ensaio" <- w58
    n144 = case shown="True" "aux_cap_ensaio" {
      tunnel: [w109 w120] -> w38
      tunnel: w43 -> [w109 w117]
      tunnel: [w108 w119] -> w39
      tunnel: w42 -> [w108 w118]
      frame False {
      }
      frame True {
        n145 = local read "Table ID"() -> (w114:u16)
        n146 = local read "cap_nom_ensaio"() -> (w112:dbl)
        n147 = call-poly <vilib>:"DB Tools Format Datetime String.vi"() -> ("date/time string"=w116:string)  [unwired: 1 in]
        n148 = local write "aux_cap_ensaio"(FALSE ("aux_cap_ensaio")) -> ()
        n149 = Bundle("Table ID"=w114, "date/time string"=w116, 0, "cap_nom_ensaio"=w112) -> (w115:T5)  [unwired: 1 in]
        n150 = call <vilib>:"DB Tools Insert Data.vi"("data"=w115, "error in (no error)"=w118, "table"="tblEnsaio", "connection reference"=w117) -> ("error out"=w119:errorcluster, "connection reference out"=w120:T4)  [unwired: 6 in]
      }
    }
    n151 = case shown="True" "aux_res_ensaio" {
      tunnel: [w90 w103] -> w34
      tunnel: w39 -> [w90 w101]
      tunnel: [w91 w104] -> w36
      tunnel: w38 -> [w91 w102]
      frame False {
      }
      frame True {
        w100 = "tblEnsaio" ("table")
        n152 = local read "Table ID"() -> (w95:u16)
        n153 = call-poly <vilib>:"DB Tools Format Datetime String.vi"() -> ("date/time string"=w94:string)  [unwired: 1 in]
        n154 = local read "res_ensaio"() -> (w93:dbl)
        n155 = local write "aux_res_ensaio"(FALSE ("aux_res_ensaio")) -> ()
        n156 = local read "curto_ensaio"() -> (w92:dbl)
        n157 = Bundle("Table ID"=w95, "date/time string"=w94, 1, "res_ensaio"=w93) -> (w98:T6)  [unwired: 1 in]
        n158 = call <vilib>:"DB Tools Insert Data.vi"("data"=w98, "error in (no error)"=w101, "table"=w100, "connection reference"=w102) -> ("error out"=w106:errorcluster, "connection reference out"=w105:T4)  [unwired: 6 in]
        n159 = Bundle("Table ID"=w95, "date/time string"=w94, 2, "curto_ensaio"=w92) -> (w99:T7)  [unwired: 1 in]
        n160 = call <vilib>:"DB Tools Insert Data.vi"("data"=w99, "error in (no error)"=w106, "table"=w100, "connection reference"=w105) -> ("error out"=w103:errorcluster, "connection reference out"=w104:T4)  [unwired: 6 in]
      }
    }
    n161 = Or(x="aux_soc_ensaio1", y="aux_soc_ensaio2") -> (x .or. y?=w33:bool)
    n162 = case shown="True" w33 {
      tunnel: [w75 w87] -> w37
      tunnel: w36 -> [w75 w85]
      tunnel: [w74 w86] -> w35
      tunnel: w34 -> [w74 w84]
      frame False {
      }
      frame True {
        n163 = local read "Table ID"() -> (w82:u16)
        n164 = local read "soc_ensaio"() -> (w77:dbl)
        n165 = local write "aux_soc_ensaio1"(FALSE ("aux_soc_ensaio1")) -> ()
        n166 = local write "aux_soc_ensaio2"(FALSE ("aux_soc_ensaio2")) -> ()
        n167 = local write "aux_soc"(FALSE ("aux_soc")) -> ()
        n168 = Format Into String(format string="%; where idbateria=%d" ("condition"), w82) -> (resulting string=w79:string)  [unwired: 2 in, 1 out]
        n169 = Bundle("soc_ensaio"=w77) -> (w78:cluster{"soc_ensaio":dbl})  [unwired: 1 in]
        n170 = call <vilib>:"DB Tools Update Data.vi"("condition"=w79, "data"=w78, "error in (no error)"=w84, "columns"=string[] ["soc"], "table"="tblBaterias", "connection reference"=w85) -> ("error out"=w86:errorcluster, "connection reference out"=w87:T4)  [unwired: 4 in]
      }
    }
  }
  n171 = case shown="True" FALSE {
    tunnel: w23 -> [w275 w280]
    tunnel: w20 -> [w276 w279]
    tunnel: [w275 w278] -> w22
    tunnel: [w276 w277] -> w21
    frame False {
    }
    frame True {
      n172 = while {
        tunnel: w279 -> [w296]
        tunnel: w280 -> [w297]
        tunnel: [w320] -> w277
        tunnel: [w319] -> w278
        shift-right: ["Output On (T)"] -> _
        shift-left: _ -> [w316]
        shift-right: [w292] -> _
        shift-left: _ -> [w291]
        stop <- FALSE stop-if-true
        # "To do list:\nOK - Generalizar o estado de carga\nOK - Generalizar o sinal de parada de recarga\nAtualizar o SOC no banco de dados\nTestar o programa com a fonte novamente\nAjustar as instruções"
        n173 = local read "Output_Current"() -> (w290:dbl)
        n174 = Get Date/Time In Seconds() -> (seconds since 1Jan1904=w292:timestamp)
        n175 = Subtract(x=w292, y=w291) -> (x-y=w289:dbl)
        n176 = local read "corrente_res"() -> (w284:dbl)
        n177 = local read "Tensao_carga"() -> (w281:dbl)
        n178 = local read "Output_Current"() -> (w308:dbl)
        n179 = Multiply(x=w289, y=w290) -> (x*y=w287:dbl)
        n180 = local read "Output_Voltage"() -> (w309:dbl)
        n181 = case shown="True" "auxiliar 2" {
          tunnel: w287 -> [w323 _]
          frame True {
            n182 = local read "Cap_nom"() -> (w327:dbl)
            n183 = Divide(x=w323, y=3600.0) -> (x/y=w321:dbl)
            n184 = Divide(x=w321, y=w327) -> (x/y=w326:dbl)
            n185 = local read "SoC_charge"() -> (w325:dbl)
            n186 = Add(x=w326, y=w325) -> (x+y=w324:dbl)
            n187 = local write "SoC_charge"(w324) -> ()
          }
          frame False {
            n188 = local read "SOC"() -> (→"SoC_charge":dbl)
          }
        }
        n189 = case shown="\"Carga TC\"" "Radio Buttons" {
          tunnel: [w330 w347] -> w299
          tunnel: [w331 w348] -> w298
          tunnel: w297 -> [w333 w346]
          tunnel: w296 -> [w332 w345]
          tunnel: "Output On (T)" -> [w329 w344]
          frame "Carga TC" {
            n190 = case shown="False" w329 {
              tunnel: w333 -> [w335 w339]
              tunnel: w332 -> [w334 w342]
              tunnel: [w334 w341] -> w330
              tunnel: [w335 w340] -> w331
              frame True {
              }
              frame False {
                n191 = local read "corrente_max"() -> (w336:dbl)
                n192 = local read "Tensao_carga"() -> (w337:dbl)
                n193 = local write "Current_Limit"(w336) -> ()
                n194 = local write "Voltage_Limit"(w337) -> ()
                n195 = call <instrlib>:"N5700 Config Voltage Limit.vi"("error"=w342, "Volt Limit"=w337, "VISA"=w339) -> ("error out"=w343:errorcluster, "VISA out"=w338:refnum<visa-resource-name>)  [unwired: 4 in]
                n196 = call <instrlib>:"N5700 Config Current Limit.vi"("error"=w343, "Current Limit"=w336, "VISA"=w338) -> ("error out"=w341:errorcluster, "VISA out"=w340:refnum<visa-resource-name>)  [unwired: 4 in]
              }
            }
          }
          frame "Carga CC" {
            n197 = case shown="False" w344 {
              tunnel: w346 -> [w350 w356]
              tunnel: w345 -> [w349 w359]
              tunnel: [w349 w358] -> w347
              tunnel: [w350 w357] -> w348
              frame True {
              }
              frame False {
                n198 = local read "Tensao_carga"() -> (w353:dbl)
                n199 = local read "corrente_max"() -> (w354:dbl)
                n200 = local write "Current_Limit"(w354) -> ()
                n201 = Multiply(x=w353, y=1.5) -> (x*y=w351:dbl)
                n202 = local write "Voltage_Limit"(w351) -> ()
                n203 = call <instrlib>:"N5700 Config Voltage Limit.vi"("error"=w359, "Volt Limit"=w351, "VISA"=w356) -> ("error out"=w360:errorcluster, "VISA out"=w355:refnum<visa-resource-name>)  [unwired: 4 in]
                n204 = call <instrlib>:"N5700 Config Current Limit.vi"("error"=w360, "Current Limit"=w354, "VISA"=w355) -> ("error out"=w358:errorcluster, "VISA out"=w357:refnum<visa-resource-name>)  [unwired: 4 in]
              }
            }
          }
        }
        n205 = Less?(x=w308, y=w284) -> (x < y?=w306:bool)
        n206 = Multiply(x=w281, y=0.95) -> (x*y=w282:dbl)
        n207 = Exclusive Or(1:w316, 2:"Output On (T)") -> (0:w312:bool)
        n208 = Not(x="Output On (T)") -> (.not. x?=w313:bool)
        n209 = Greater?(x=w309, y=w282) -> (0:w307:bool)
        n210 = And(x="Output On (T)", y=w312) -> (x .and. y?=w315:bool)
        n211 = And(x=w313, y=w312) -> (x .and. y?=w314:bool)
        n212 = And(x=w307, y=w306) -> (x .and. y?=w301:bool)
        n213 = case shown="True" w315 {
          selector: w315 -> [_ w377]
          tunnel: w299 -> [w376 w382]
          tunnel: w298 -> [w375 w378]
          tunnel: [w376 w381] -> w311
          tunnel: [w375 w379] -> w310
          frame False {
          }
          frame True {
            n214 = local write "auxiliar 2"(w377) -> ()
            n215 = call <instrlib>:"N5700 Config Output On-Off.vi"("error"=w382, "Output ON"=TRUE, "VISA"=w378) -> ("error out"=w381:errorcluster, "VISA out"=w379:refnum<visa-resource-name>)  [unwired: 4 in]
          }
        }
        n216 = case shown="True" w314 {
          tunnel: w311 -> [w368 w374]
          tunnel: w310 -> [w369 w373]
          tunnel: [w369 w372] -> w304
          tunnel: [w368 w371] -> w305
          frame False {
          }
          frame True {
            n217 = call <instrlib>:"N5700 Config Output On-Off.vi"("error"=w374, "Output ON"=FALSE, "VISA"=w373) -> ("error out"=w371:errorcluster, "VISA out"=w372:refnum<visa-resource-name>)  [unwired: 4 in]
          }
        }
        n218 = case shown="True" w301 {
          tunnel: w305 -> [w362 w367]
          tunnel: w304 -> [w361 w365]
          tunnel: [w362 w366] -> w303
          tunnel: [w361 w364] -> w302
          frame False {
          }
          frame True {
            w363 = FALSE ("Output ON")
            n219 = local write "Output On (T)"(w363) -> ()
            n220 = call <instrlib>:"N5700 Config Output On-Off.vi"("error"=w367, "Output ON"=w363, "VISA"=w365) -> ("error out"=w366:errorcluster, "VISA out"=w364:refnum<visa-resource-name>)  [unwired: 4 in]
          }
        }
        n221 = call <instrlib>:"N5700 Meas Output Voltage.vi"("error"=w303, "VISA"=w302) -> ("error out"=w318:errorcluster, "Output Voltage"=→"Waveform Chart Voltage" →"Output_Voltage":dbl, "VISA out"=w317:refnum<visa-resource-name>)  [unwired: 4 in]
        n222 = call <instrlib>:"N5700 Meas Output Current.vi"("error"=w318, "VISA"=w317) -> ("error out"=w320:errorcluster, "Output Current"=→"Waveform Chart Current" →"Output_Current":dbl, "VISA out"=w319:refnum<visa-resource-name>)  [unwired: 4 in]
        "Charge Active" <- "Output On (T)"
        "Status_PS" <- TRUE ("Status_PS")
        "Status_output_DC 2" <- "Output On (T)"
      }
    }
  }
  n223 = call <instrlib>:"N5700 Close.vi"("error"=w21, "VISA name"=w22) -> ("error out"=→"error out":errorcluster)  [unwired: 6 in]
  n224 = case shown="True" FALSE {
    frame False {
    }
    frame True {
      n225 = call <instrlib>:"Initialize NHRDCLoad.vi"("reset device (Off)"=TRUE, "resource name"=refnum<visa-resource-name> "DC Load 2") -> ("error out"=w384:errorcluster, "instrument handle out"=w383:refnum<visa-resource-name>)  [unwired: 8 in]
      n226 = call <instrlib>:"Get Current Range.vi"("error in (no error)"=w384, "instrument handle"=w383) -> ("error out"=w386:errorcluster, "instrument handle out"=w385:refnum<visa-resource-name>)  [unwired: 7 in, 1 out]
      n227 = while {
        tunnel: [w417] -> w388
        tunnel: [w416] -> w387
        tunnel: w386 -> [w415]
        tunnel: w385 -> [w414]
        shift-right: [w407] -> _
        shift-left: _ -> [w406]
        shift-right: [w397] -> _
        shift-left: _ -> [w401]
        stop <- FALSE stop-if-true
        w422 = u16 3 items=["AC + DC Current", "AC + DC Voltage", "DC Current", "DC Voltage", "First 10% Current", "First 10% Voltage", "Last 10% Current", "Last 10% Voltage", "Negative Peak Current", "Negative Peak Voltage", "Positive Peak Current", "Positive Peak Voltage", "Average Power", "Resistance", "RMS Current", "RMS Voltage"] ("Measurement")
        w421 = u16 2 items=["AC + DC Current", "AC + DC Voltage", "DC Current", "DC Voltage", "First 10% Current", "First 10% Voltage", "Last 10% Current", "Last 10% Voltage", "Negative Peak Current", "Negative Peak Voltage", "Positive Peak Current", "Positive Peak Voltage", "Average Power", "Resistance", "RMS Current", "RMS Voltage"] ("Measurement")
        w420 = 1 items=["NHRDCLOAD_VAL_LOAD_MODE_OFF"=0, "NHRDCLOAD_VAL_LOAD_MODE_CC"=1, "NHRDCLOAD_VAL_LOAD_MODE_CR"=2, "NHRDCLOAD_VAL_LOAD_MODE_CV"=4, "NHRDCLOAD_VAL_LOAD_MODE_CP"=8, "NHRDCLOAD_VAL_LOAD_MODE_XCC"=16, "NHRDCLOAD_VAL_LOAD_MODE_LED"=32, "NHRDCLOAD_VAL_LOAD_MODE_MPPT"=64, "NHRDCLOAD_VAL_LOAD_MODE_XY"=128, "NHRDCLOAD_VAL_LOAD_MODE_SC"=32768] ("active mode")
        # "To do list:\nAjustar as instruções de ensaios\nOK - Atualizar o SOC no banco de dados\nColocar mensagem de aprovado ou recusado no ensaio\nAuxiliar SOC ainda ativo sem o banco de dados - arrumar"
        n228 = local read "Status_output_DC"() -> (w405:bool)
        n229 = local read "Ensaios"() -> (w413:u16)
        n230 = Get Date/Time In Seconds() -> (seconds since 1Jan1904=w407:timestamp)
        n231 = Subtract(x=w407, y=w406) -> (x-y=w403:dbl)
        n232 = case shown="0, Default" w413 {
          tunnel: [w442 "corr_fn" w479 0.0 ("corr_fn") "curr_carac"] -> w412
          tunnel: [w439 w456 w480 TRUE ("y") w540] -> w410
          frame 0, Default {
            # "To do list\nOK - Colocar botao para desativar o banco de dados\nOK - Implementar o baco de dados\nOK - Generalizar a tensao de corte\nOK - Inserir no banco de dados os resultados"
            n233 = local read "padrao_cap"() -> (w436:dbl)
            "padrao_cap2" <- w436
            n234 = local read "Timer_ensaio"() -> (w441:dbl)
            n235 = local read "Cap_nom"() -> (w437:dbl)
            "cap_bat" <- w437
            n236 = Greater?(x=w441, y=0.0) -> (0:w438:bool)
            n237 = case shown="True" w438 {
              tunnel: [FALSE ("COP") TRUE ("COP")] -> w439
              frame False {
              }
              frame True {
                # "To do list:\nSinal para escrever o soc no banco de dados"
                n238 = local read "DC_Voltage"() -> (w449:dbl)
                n239 = local read "Tensao_corte"() -> (w445:dbl)
                n240 = local read "cap_ensaio"() -> (→"cap_nom_ensaio":dbl)
                n241 = Greater?(x=w449, y=w445) -> (0:w448:bool)
                n242 = case shown="False" w448 {
                  frame False {
                    n243 = local read "Ativar Banco"() -> (w450:bool)
                    n244 = local write "aux_cap_ensaio"(TRUE ("aux_cap_ensaio")) -> ()
                    n245 = local write "Start"(FALSE ("Start")) -> ()
                    n246 = case shown="False" w450 {
                      frame False {
                        n247 = local read "soc_ensaio"() -> (w453:dbl)
                        n248 = local write "SOC"(w453) -> ()
                      }
                      frame True {
                        n249 = local write "aux_soc_ensaio1"(TRUE ("aux_soc_ensaio1")) -> ()
                      }
                    }
                  }
                  frame True {
                  }
                }
                n250 = local write "aux_soc"(TRUE ("aux_soc")) -> ()
              }
            }
            n251 = Divide(x=w437, y=w436) -> (x/y=w442:dbl)
            n252 = local write "cap_soc"(w437) -> ()
          }
          frame 1 {
            # "To do list:\nOK - Generalizar a tensao de corte"
            n253 = local write "cap_soc"("cap_fn") -> ()
            n254 = local read "Timer_ensaio"() -> (w459:dbl)
            n255 = Greater?(x=w459, y=0.0) -> (0:w457:bool)
            n256 = case shown="True" w457 {
              tunnel: [FALSE ("y") TRUE ("y")] -> w456
              frame False {
              }
              frame True {
                n257 = local read "Tensao_corte"() -> (w463:dbl)
                n258 = local read "DC_Voltage"() -> (w467:dbl)
                n259 = local read "cap_ensaio"() -> (→"cap_fn_calc":dbl)
                n260 = Greater?(x=w467, y=w463) -> (0:w465:bool)
                n261 = local write "aux_soc"(TRUE ("aux_soc")) -> ()
                n262 = case shown="False" w465 {
                  frame False {
                    n263 = local read "Ativar Banco"() -> (w468:bool)
                    n264 = local write "aux_soc"(FALSE ("aux_soc")) -> ()
                    n265 = local write "Start"(FALSE ("Start")) -> ()
                    n266 = case shown="False" w468 {
                      frame False {
                        n267 = local read "soc_ensaio"() -> (w471:dbl)
                        n268 = local write "SOC"(w471) -> ()
                      }
                      frame True {
                        n269 = local write "aux_soc_ensaio2"(TRUE ("aux_soc_ensaio2")) -> ()
                      }
                    }
                  }
                  frame True {
                  }
                }
              }
            }
          }
          frame 2 {
            # "To do list:\nOK - Implementar um botao para desativar o banco de dados\nOK - Implementar um botao para selecionar o tipo de bateria\nOK - Inserir no banco de dados os resultados\nVer o que muda para o ensaio de baterias de litio"
            n270 = local read "Timer_ensaio"() -> (w482:dbl)
            n271 = local read "Cap_nom"() -> (w473:dbl)
            "res_cap" <- w473
            n272 = To Long Integer(number=w482) -> (32bit integer=w481:i32)
            n273 = case shown="326..330" w481 {
              tunnel: [FALSE ("y") TRUE ("y") FALSE ("y") TRUE ("y") FALSE ("y")] -> w480
              tunnel: [1.0 ("y") 1.0 ("y") 1.0 ("y") 5.0 ("y") 5.0 ("y")] -> w478
              frame 0, Default {
              }
              frame 1..20 {
                n274 = local read "DC_Voltage"() -> (→"res_volt_1":dbl)
                n275 = local read "DC_Current"() -> (→"res_curr_1":dbl)
                n276 = local write "aux_soc"(TRUE ("aux_soc")) -> ()
              }
              frame 21..320 {
              }
              frame 321..325 {
                n277 = local read "DC_Voltage"() -> (→"res_volt_2":dbl)
                n278 = local read "DC_Current"() -> (→"res_curr_2":dbl)
              }
              frame 326..330 {
                n279 = local read "Ativar Banco"() -> (w496:bool)
                n280 = local read "res_volt_2"() -> (w505:dbl)
                n281 = local read "res_curr_1"() -> (w506:dbl)
                n282 = local read "res_volt_1"() -> (w507:dbl)
                n283 = local read "res_volt_2"() -> (w508:dbl)
                n284 = local read "res_volt_1"() -> (w514:dbl)
                n285 = local read "res_curr_2"() -> (w516:dbl)
                n286 = local read "res_curr_1"() -> (w513:dbl)
                n287 = local read "res_volt_2"() -> (w515:dbl)
                n288 = local read "res_volt_1"() -> (w503:dbl)
                n289 = local read "res_curr_2"() -> (w504:dbl)
                n290 = local write "Start"(FALSE ("Start")) -> ()
                n291 = local write "aux_res_ensaio"(TRUE ("aux_res_ensaio")) -> ()
                n292 = Subtract(x=w507, y=w508) -> (x-y=w500:dbl)
                n293 = Multiply(x=w505, y=w506) -> (x*y=w502:dbl)
                n294 = Multiply(x=w503, y=w504) -> (x*y=w501:dbl)
                n295 = Subtract(x=w516, y=w513) -> (x-y=w512:dbl)
                n296 = Subtract(x=w514, y=w515) -> (x-y=w511:dbl)
                n297 = case shown="False" w496 {
                  frame False {
                    n298 = local read "soc_ensaio"() -> (w519:dbl)
                    n299 = local write "SOC"(w519) -> ()
                  }
                  frame True {
                    n300 = local write "aux_soc_ensaio2"(TRUE ("aux_soc_ensaio2")) -> ()
                  }
                }
                n301 = Subtract(x=w501, y=w502) -> (x-y=w499:dbl)
                n302 = Divide(x=w511, y=w512) -> (x/y=→"res_ensaio":dbl)
                n303 = Divide(x=w499, y=w500) -> (x/y=→"curto_ensaio":dbl)
              }
            }
            n304 = Divide(x=w473, y=10.0) -> (x/y=w476:dbl)
            n305 = Multiply(x=w476, y=4.0) -> (x*y=w475:dbl)
            n306 = local write "cap_soc"(w473) -> ()
            n307 = Multiply(x=w475, y=w478) -> (x*y=w479:dbl)
          }
          frame 3 {
            # "To do list:\nImplementar o codigo para realizar o ensaio ciclico"
          }
          frame 4 {
            n308 = local read "Start"() -> (w531:bool)
            n309 = local read "Timer_ensaio"() -> (w554:dbl)
            n310 = local read "pulso_soc"() -> (w524:dbl)
            n311 = local read "cont_pulso"() -> (w535:dbl)
            n312 = Divide(x=100.0 ("y"), y=w524) -> (x/y=w529:dbl)
            n313 = case shown="True" w531 {
              frame False {
              }
              frame True {
                # "To do list:\nGeneralizar a aquisição de dados\nEnviar corrente drenada, numero de pulsos, variação do SOC\nCampo para dar um nome e criar uma pasta e escolher o nome do arquivo"
                n314 = local read "DC_Current"() -> (w555:dbl)
                n315 = local read "DC_Voltage"() -> (w557:dbl)
                n316 = local read "Timer_ensaio"() -> (w558:dbl)
                n317 = Build Array(w555) -> (w556:dbl[])
                n318 = Build Array(w557) -> (w560:dbl[])
                n319 = Build Array(w558) -> (w559:dbl[])
                n320 = call-poly <vilib>:"Write Delimited Spreadsheet.vi"("file path (dialog if empty)"=path "C:/Users/Pichau/Desktop/William Rocha/Projeto Integrador - William Rocha/caracterizacao/data_current.csv", "1D data"=w556, "append to file? (new file:F)"=TRUE) -> ()  [unwired: 11 in, 2 out]
                n321 = call-poly <vilib>:"Write Delimited Spreadsheet.vi"("file path (dialog if empty)"=path "C:/Users/Pichau/Desktop/William Rocha/Projeto Integrador - William Rocha/caracterizacao/data_voltage.csv", "1D data"=w560, "append to file? (new file:F)"=TRUE) -> ()  [unwired: 11 in, 2 out]
                n322 = call-poly <vilib>:"Write Delimited Spreadsheet.vi"("file path (dialog if empty)"=path "C:/Users/Pichau/Desktop/William Rocha/Projeto Integrador - William Rocha/caracterizacao/data_timer.csv", "1D data"=w559, "append to file? (new file:F)"=TRUE) -> ()  [unwired: 11 in, 2 out]
              }
            }
            n323 = Greater?(x=w554, y="tinicio") -> (0:w552:bool)
            n324 = Add(x=w529, y=1.0) -> (x+y=w528:dbl)
            n325 = case shown="True" w552 {
              frame False {
              }
              frame True {
                n326 = local read "COP"() -> (w572:bool)
                n327 = case shown="False" w572 {
                  frame False {
                    n328 = local read "cont_pulso"() -> (w574:dbl)
                    n329 = local write "COP"(TRUE ("COP")) -> ()
                    n330 = local read "tpulso"() -> (w578:dbl)
                    n331 = local read "tinicio"() -> (w577:dbl)
                    n332 = Add(x=1.0, y=w574) -> (x+y=→"cont_pulso":dbl)
                    n333 = Add(x=w577, y=w578) -> (x+y=w579:dbl)
                    n334 = local write "tinicio"(w579) -> ()
                  }
                  frame True {
                    n335 = local read "tinicio"() -> (w581:dbl)
                    n336 = local read "twait"() -> (w582:dbl)
                    n337 = Add(x=w581, y=w582) -> (x+y=w583:dbl)
                    n338 = local write "tinicio"(w583) -> ()
                    n339 = local write "COP"(FALSE ("COP")) -> ()
                  }
                }
              }
            }
            n340 = Greater Or Equal?(x=w535, y=w528) -> (x >= y?=w539:bool)
            n341 = case shown="True" w539 {
              frame False {
              }
              frame True {
                n342 = local write "Start"(FALSE ("Start")) -> ()
              }
            }
            n343 = Divide(x="pulso_soc", y=100.0) -> (x/y=w546:dbl)
            n344 = local read "curr_carac"() -> (w545:dbl)
            n345 = Multiply(x="cap_caract", y=w546) -> (x*y=w542:dbl)
            n346 = local read "Start"() -> (w549:bool)
            n347 = local write "cap_soc"("cap_caract") -> ()
            n348 = Divide(x=w542, y=w545) -> (x/y=w544:dbl)
            n349 = Not(x=w549) -> (.not. x?=w550:bool)
            n350 = Multiply(x=w544, y=3600.0) -> (x*y=w537:dbl)
            "tpulso" <- w537
            n351 = case shown="True" w550 {
              frame False {
                n352 = local write "aux_soc"(TRUE ("aux_soc")) -> ()
              }
              frame True {
                n353 = local write "COP"(FALSE ("COP")) -> ()
                n354 = local write "cont_pulso"(0.0 ("cont_pulso")) -> ()
                n355 = local write "tinicio"(5.0 ("twait")) -> ()
              }
            }
            n356 = local read "pulso_soc"() -> (w525:dbl)
            n357 = Add(x="twait", y=w537) -> (x+y=w536:dbl)
            n358 = Divide(x=100.0 ("y"), y=w525) -> (x/y=w530:dbl)
            n359 = Multiply(x=w536, y=w530) -> (x*y=w534:dbl)
            n360 = Add(x=w534, y=5.0) -> (x+y=→"est_time":dbl)
            n361 = local read "COP"() -> (w540:bool)
          }
        }
        n362 = local write "info_ensaio"(w413) -> ()
        n363 = case shown="True" w405 {
          tunnel: [0.0 ("DC_Current") w435] -> w404
          frame False {
          }
          frame True {
            n364 = local read "DC_Current"() -> (w435:dbl)
          }
        }
        n365 = Multiply(x=w403, y=w404) -> (x*y=w399:dbl)
        n366 = Divide(x=w399, y=3600.0) -> (x/y=w394:dbl)
        n367 = Add(x=w394, y=w401) -> (x+y=w402:dbl)
        n368 = local read "Start"() -> (w400:bool)
        n369 = Select(t=w402, s=w400, f=0.0) -> (s? t:f=w397:dbl)
        "cap_ensaio" <- w397
        n370 = case shown="True" "aux_soc" {
          tunnel: w394 -> [_ w433]
          frame False {
            n371 = local read "SOC"() -> (w426:dbl)
            n372 = local write "soc_ensaio"(w426) -> ()
          }
          frame True {
            n373 = Divide(x=w433, y="cap_soc") -> (x/y=w429:dbl)
            n374 = local read "soc_ensaio"() -> (w431:dbl)
            n375 = Multiply(x=w429, y=100.0) -> (x*y=w427:dbl)
            n376 = Subtract(x=w431, y=w427) -> (x-y=→"soc_ensaio":dbl)
          }
        }
        n377 = Not(x="Start") -> (.not. x?=w391:bool)
        n378 = And(x="Start", y=w410) -> (x .and. y?=w409:bool)
        "Status_output_DC" <- w409
        n379 = property on="Ensaios" class="Ring (strict)"("Visible"=w391) -> ()  [unwired: 2 in, 2 out]
        n380 = call <instrlib>:"Set Current Enabled.vi"("error in (no error)"=w415, "current enabled (false)"=w409, "instrument handle"=w414) -> ()  [unwired: 7 in, 2 out]
        n381 = call <instrlib>:"Set Current.vi"("error in (no error)"=w415, "current (0.0)"=w412, "instrument handle"=w414) -> ()  [unwired: 7 in, 2 out]
        n382 = call <instrlib>:"Get Active Mode.vi"("error in (no error)"=w415, "instrument handle"=w414) -> ("active mode"=w419:i32)  [unwired: 7 in, 2 out]
        n383 = call <instrlib>:"Read.vi"("error in (no error)"=w415, "max time milliseconds (infinite)"=100, "measurement (NHRDCLOAD_VAL_MEASURE_AC_PLUS_DC_CURRENT)"=w421, "instrument handle"=w414) -> ("measured value"=→"DC_Current" →"WFC Current Load":dbl)  [unwired: 5 in, 2 out]
        n384 = call <instrlib>:"Read.vi"("error in (no error)"=w415, "max time milliseconds (infinite)"=100, "measurement (NHRDCLOAD_VAL_MEASURE_AC_PLUS_DC_CURRENT)"=w422, "instrument handle"=w414) -> ("error out"=w416:errorcluster, "measured value"=→"DC_Voltage" →"WFC Voltage Load":dbl, "instrument handle out"=w417:refnum<visa-resource-name>)  [unwired: 5 in]
        n385 = Equal?(x=w419, y=w420) -> (x = y?=→"CC Active":bool)
        "Status_DC" <- TRUE ("Status_DC")
      }
      n386 = call <instrlib>:"Close NHRDCLoad.vi"("error in (no error)"=w387, "instrument handle"=w388) -> ()  [unwired: 9 in, 1 out]
    }
  }
  n387 = call <vilib>:"DB Tools Close Connection.vi"("error in (no error)"=w4, "connection reference"=w5) -> ()  [unwired: 5 in, 1 out]
